vi "Read Profile.vi"(8 "error in":errorcluster, 10 "Name":string, 11 "File in":T1) -> (0 "error out":errorcluster, 2 "Profile":T2, 3 "File out":T1)   [LabVIEW 2025, in "TS Environment Manager.lvlib"]
doc: "This VI retrieves a profile from the provided file by its name. If the profile does not exist the vi produces an error."
uses:
  TS Environment Manager.lvlib
  <vilib>/Utility/config.llb/Config Data RefNum.ctl
  Type Definitions/Profile--cluster.ctl
  Type Definitions/Architecture--enum.ctl
  <vilib>/Utility/config.llb/Read Key (String).vi
  <vilib>/Utility/config.llb/Read Key (Path).vi
  <vilib>/Utility/config.llb/NI_LVConfig.lvlib
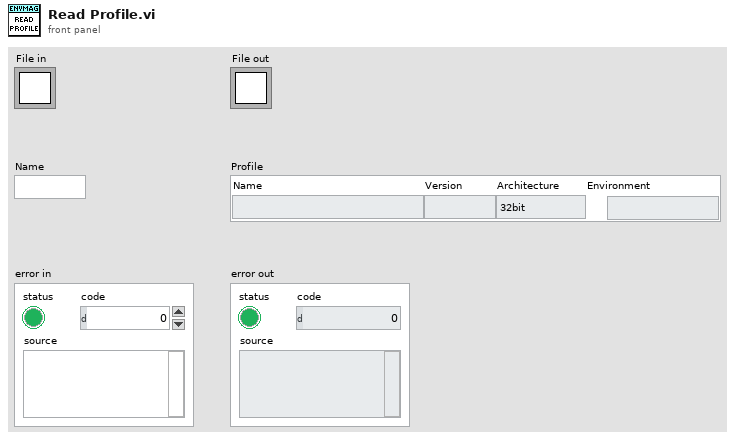
[diagram p1: front panel]
types:
  T1 = typedef "NI_LVConfig.lvlib/Config Data RefNum.ctl" = refnum<k1>
  T2 = typedef "Profile--cluster.ctl" = cluster{"Name":string, "Version":string, "Architecture":T3, "Environment":path}
  T3 = typedef "Architecture--enum.ctl" = enum16{"32bit", "64bit"}
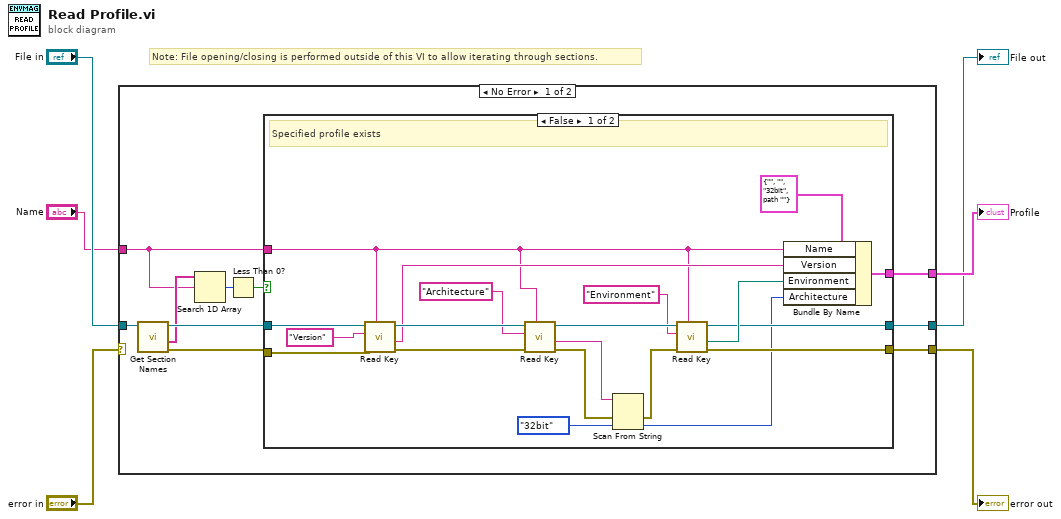
[diagram p0: block diagram]
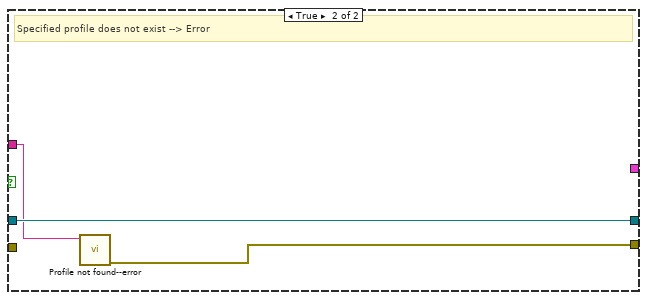
[diagram p2: hidden frame]
diagram:
  # "Note: File opening/closing is performed outside of this VI to allow iterating through sections."
  n1 = case shown="No Error" "error in" {
    selector: "error in" -> [_ w41]
    tunnel: "File in" -> [w13 w40]
    tunnel: "Name" -> [w9 _]
    tunnel: [w16 _] -> w4
    tunnel: [w15 w41] -> w2
    tunnel: [w14 w40] -> w1
    frame No Error {
      n2 = call <vilib>:"Get Section Names.vi"("refnum"=w13) -> ("error out"=w11:errorcluster, "section names"=w10:string[], "refnum out"=w12:T1)  [unwired: 8 in]
      n3 = Search 1D Array(1D array=w10, element=w9) -> (index of element=w8:i32)  [unwired: 1 in]
      n4 = Less Than 0?(x=w8) -> (x < 0?=w7:bool)
      n5 = case shown="False" w7 {
        tunnel: [w24 _] -> w16
        tunnel: [w23 w38] -> w15
        tunnel: [w21 w39] -> w14
        tunnel: w12 -> [w19 w39]
        tunnel: w11 -> [w18 _]
        tunnel: w9 -> [w17 w37]
        frame False {
          # "Specified profile exists"
          n6 = call-poly <vilib>:"Read Key.vi"("section"=w17, "error in (no error)"=w18, "key"="Version", "refnum"=w19) -> ("error out"=w35:errorcluster, "value"=w28:string, "refnum out"=w36:T1)  [unwired: 4 in, 1 out]
          n7 = call-poly <vilib>:"Read Key.vi"("section"=w17, "error in (no error)"=w35, "key"="Architecture", "refnum"=w36) -> ("error out"=w26:errorcluster, "value"=w32:string, "refnum out"=w31:T1)  [unwired: 4 in, 1 out]
          n8 = Scan From String(input string=w32, error in=w26, default 1=Architecture--enum."32bit" ("Architecture")) -> (error out=w25:errorcluster, output 1=w20:T3)  [unwired: 2 in, 2 out]
          n9 = call-poly <vilib>:"Read Key.vi"("section"=w17, "error in (no error)"=w25, "key"="Environment", "refnum"=w31) -> ("error out"=w23:errorcluster, "value"=w27:path, "refnum out"=w21:T1)  [unwired: 4 in, 1 out]
          n10 = Bundle By Name(cluster=T2 {"Name"="", "Version"="", "Architecture"=enum."32bit", "Environment"=path ""} ("Profile"), "Name"=w17, "Version"=w28, "Environment"=w27, "Architecture"=w20) -> (w24:T2)
        }
        frame True {
          # "Specified profile does not exist --> Error"
          n11 = call "Profile not found--error.vi"("Name"=w37) -> ("error out"=w38:errorcluster)  [unwired: 10 in]
        }
      }
    }
    frame Error {
      # "Pass error without further action"
    }
  }
  "error out" <- w2
  "Profile" <- w4
  "File out" <- w1
